vi "_Debug_leer asic y fpga_enlazado.vi"(8 "error in":errorcluster, 11 "Handle":u32) -> (0 "error out":errorcluster, 3 "ftHandle_out":u32)   [LabVIEW 2009]
panel:
  out "Scaler 3 (20,21)":u16 format="%04x"
  out "Scaler 2 (18,19)":u16 format="%04x"
  out "Scaler 1 (16,17)":u16 format="%04x"
  out "Lectura asic (14,15)":u16 format="%04x"
  out "Vent. Sacaler (11,12,13)":u32 format="%06x"
  out "Periodo VGa (9,10)":u16 format="%04x"
  out "Pulse VGa (7,8)":u16 format="%04x"
  out "Ganacia VGA (6)":u8 format="%02x"
  out "adc (4,5)":u16 format="%04x"
  out "Asic (1,2,3)":u32 format="%06x"
  out "DIR 0 (CONFIG)":bool[](array[boolean])
  out "ERROR":bool
  out "UPDATE":bool
  in  "stop":bool
  out "DAC_IB":bool[](array[boolean])
  out "BUFF_ENA":bool
  out "LVDS_ENA1":bool
  out "LVDS_ENA0":bool
  out "MUX_ENA":string
  out "MUX_ENA#":i32
  out "IN 0":bool[](array[boolean])
  out "IN 6":bool[](array[boolean])
  out "IN 5":bool[](array[boolean])
  out "IN 4":bool[](array[boolean])
  out "IN 3":bool[](array[boolean])
  out "IN 2":bool[](array[boolean])
  out "IN 1":bool[](array[boolean])
  out "DAC_MUX#":i32
  out "DAC_MUX":string
  out "TH5":u16 format="%010b"
  out "TH4":u16 format="%010b"
  out "TH3":u16 format="%010b"
  out "TH2":u16 format="%010b"
  out "TH1":u16 format="%010b"
  out "TH0":u16 format="%010b"
  # "start vent. sca\nescribir ganancia\nactualizar pulso\nenable pulso\nstart tx asic\nreset asic\nescribir adc"
  # "IB5\nIB4\nIB3\nIB2\nIB1\nIB0"
  # "Control_byte\nNum bit        Función\n0            \"Escribir\" ADC\n1                      \"INIT_R\" ASIC (reset)\n2                      \"start_tx\" ASIC para configuración ASIC\n3                      \"enable\" para el pulso\n4                      \"actualizar\" para el pulso\n5                      \"Escribir_ganancia\" para configuración ganancia\n6                      \"start\" para apertura ventana temportal scalers"
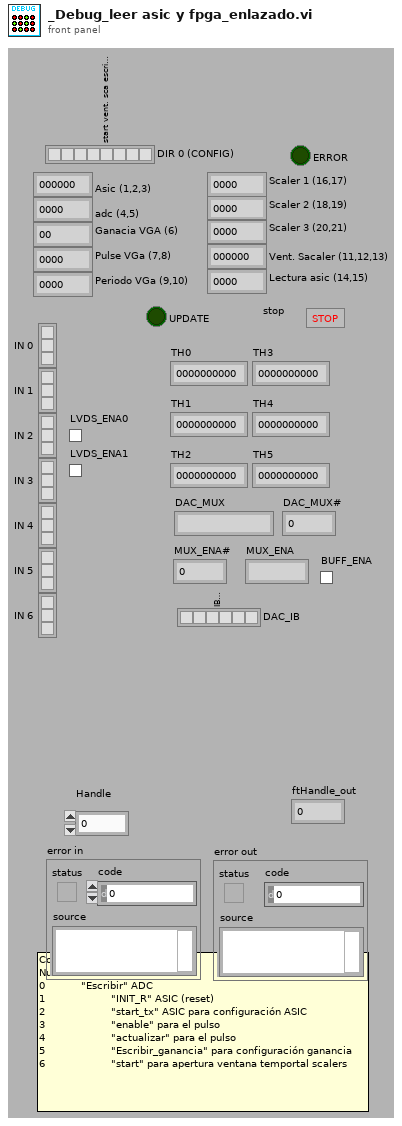
[diagram p1: front panel]
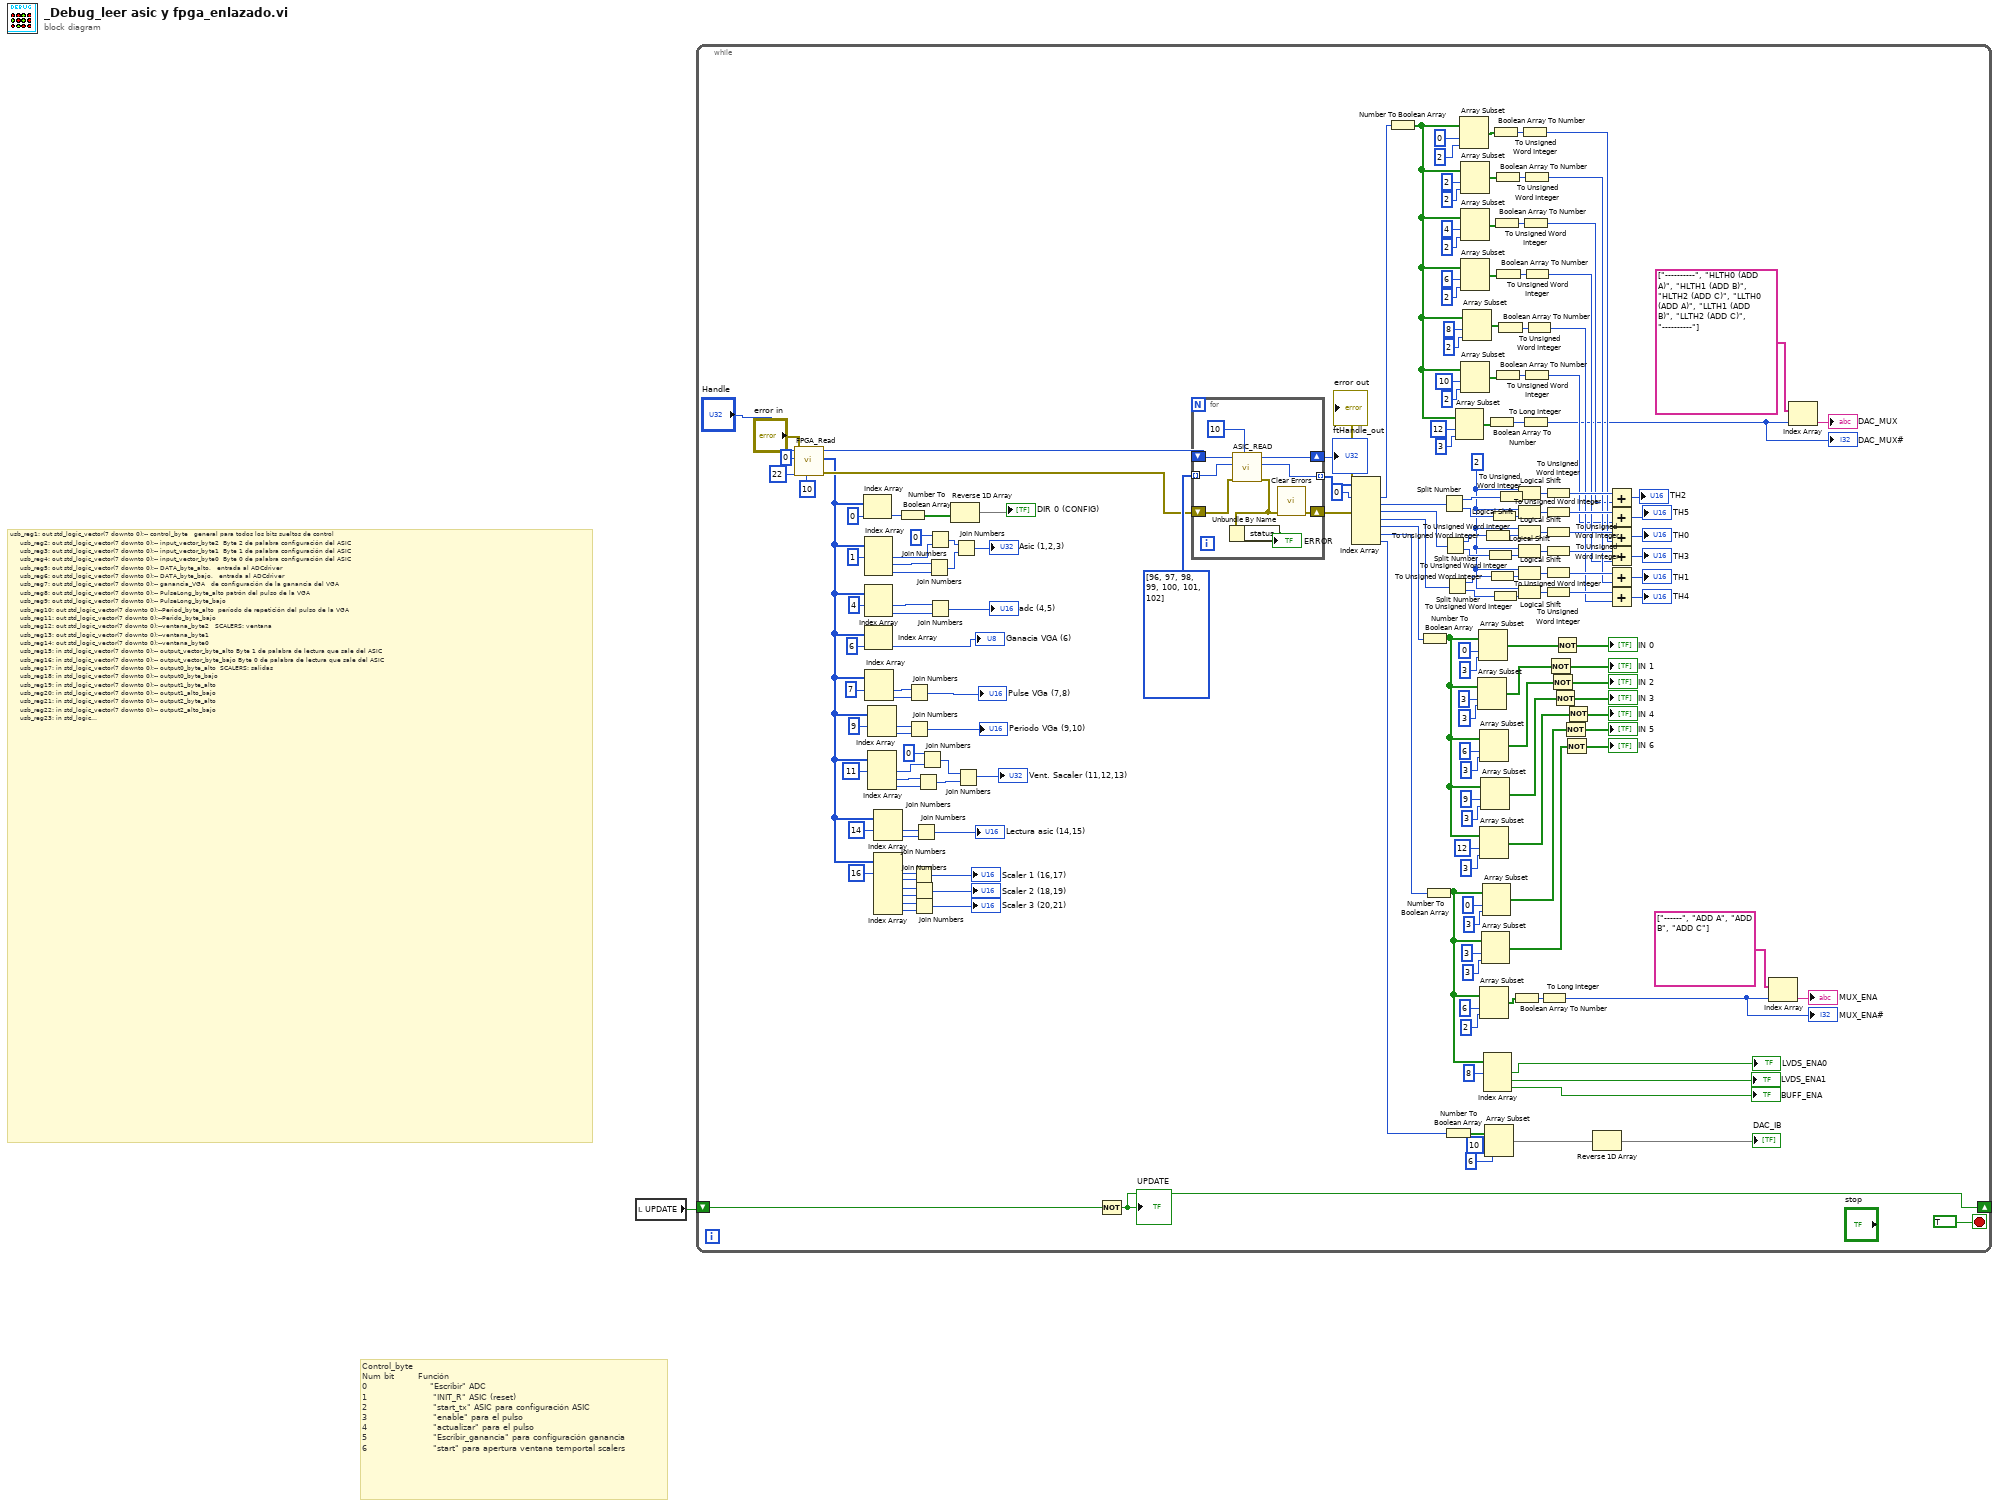
[diagram p0: block diagram]
diagram:
  # "Control_byte\nNum bit        Función\n0                     \"Escribir\" ADC\n1                      \"INIT_R\" ASIC (reset)\n2                      \"start_tx\" ASIC para configuración ASIC\n3                      \"enable\" para el pulso\n4                      \"actualizar\" para el pulso\n5                      \"Escribir_ganancia\" para configuración ganancia\n6                      \"start\" para apertura ventana temportal scalers"
  # "usb_reg1: out std_logic_vector(7 downto 0);-- control_byte\t\t\tgeneral para todos los bits sueltos de control\n\t\t\t  usb_reg2: out std_logic_vector(7 downto 0);-- input_vector_byte2 \tByte 2 de palabra configuración del ASIC\n\t\t\t  usb_reg3: out std_logic_vector(7 downto 0);-- input_vector_byte1 \tByte 1 de palabra configuración del ASIC\n\t\t\t  usb_reg4: out std_logic_vector(7 downto 0);-- input_vector_byte0 \tByte 0 de palabra configuración del ASIC\n\t\t\t  usb_reg5: out std_logic_vector(7 downto 0);-- DATA_byte_alto, \t\tentrada al ADCdriver\n\t\t\t  usb_reg6: out std_logic_vector(7 downto 0);-- DATA_byte_bajo, \t\tentrada al ADCdriver\n\t\t\t  usb_reg7: out std_logic_vector(7 downto 0);-- ganancia_VGA\t\t\tde configuración de la ganancia del VGA\n\t\t\t  usb_reg8: out std_logic_vector(7 downto 0);-- PulseLong_byte_alto\tpatrón del pulso de la VGA\n\t\t\t  usb_reg9: out std_logic_vector(7 downto 0);-- PulseLong_byte_bajo\n\t\t\t  usb_reg10: out std_logic_vector(7 downto 0);--Period_byte_alto\t\tperíodo de repetición del pulso de la VGA\n\t\t\t  usb_reg11: out std_logic_vector(7 downto 0);--Perido_byte_bajo\n\t\t\t  usb_reg12: out std_logic_vector(7 downto 0);--ventana_byte2\t\t\tSCALERS: ventana\n\t\t\t  usb_reg13: out std_logic_vector(7 downto 0);--ventana_byte1\t\n\t\t\t  usb_reg14: out std_logic_vector(7 downto 0);--ventana_byte0\n\t\t\t  usb_reg15: in std_logic_vector(7 downto 0);-- output_vector_byte_alto\tByte 1 de palabra de lectura que sale del ASIC\n\t\t\t  usb_reg16: in std_logic_vector(7 downto 0);-- output_vector_byte_bajo\tByte 0 de palabra de lectura que sale del ASIC\n\t\t\t  usb_reg17: in std_logic_vector(7 downto 0);-- output0_byte_alto\t\tSCALERS: salidas\n\t\t\t  usb_reg18: in std_logic_vector(7 downto 0);-- output0_byte_bajo\n\t\t\t  usb_reg19: in std_logic_vector(7 downto 0);-- output1_byte_alto\n\t\t\t  usb_reg20: in std_logic_vector(7 downto 0);-- output1_alto_bajo \n\t\t\t  usb_reg21: in std_logic_vector(7 downto 0);-- output2_byte_alto \n\t\t\t  usb_reg22: in std_logic_vector(7 downto 0);-- output2_alto_bajo \n\t\t\t  usb_reg23: in std_logic_vector(7 downto 0);-- para el canal_0 del ADCdriver\n\t\t\t  usb_reg24: in std_logic_vector(7 downto 0);\n\t\t\t  usb_reg25: in std_logic_vector(7 downto 0);-- para el canal_1 del ADCdriver\n\t\t\t  usb_reg26: in std_logic_vector(7 downto 0);\n\t\t\t  usb_reg27: in std_logic_vector(7 downto 0);-- para el canal_2 del ADCdriver\n\t\t\t  usb_reg28: in std_logic_vector(7 downto 0);\n\t\t\t  usb_reg29: in std_logic_vector(7 downto 0);-- para el canal_3 del ADCdriver\n\t\t\t  usb_reg30: in std_logic_vector(7 downto 0);\n\t\t\t  usb_reg31: in std_logic_vector(7 downto 0);-- para el canal_4 del ADCdriver\n\t\t\t  usb_reg32: in std_logic_vector(7 downto 0);\n\t\t\t  usb_reg33: in std_logic_vector(7 downto 0);-- para el canal_5 del ADCdriver\n\t\t\t  usb_reg34: in std_logic_vector(7 downto 0);\n\t\t\t  usb_reg35: in std_logic_vector(7 downto 0);-- para el canal_6 del ADCdriver\n\t\t\t  usb_reg36: in std_logic_vector(7 downto 0);\n\t\t\t  usb_reg37: in std_logic_vector(7 downto 0);-- para el canal_7 del ADCdriver\n\t\t\t  usb_reg38: in std_logic_vector(7 downto 0);\n\t\t\t  usb_reg39: in std_logic_vector(7 downto 0);-- para el canal_8 del ADCdriver\n\t\t\t  usb_reg40: in std_logic_vector(7 downto 0);\n\t\t\t  usb_reg41: in std_logic_vector(7 downto 0);-- para el canal_9 del ADCdriver\n\t\t\t  usb_reg42: in std_logic_vector(7 downto 0);\n\t\t\t  usb_reg43: in std_logic_vector(7 downto 0);-- para el canal_10 del ADCdriver\n\t\t\t  usb_reg44: in std_logic_vector(7 downto 0)--;"
  n1 = local read "UPDATE"() -> (w1:bool)
  n2 = while {
    shift-right: [w76] -> _
    shift-left: w1 -> [w14]
    stop <- TRUE stop-if-true
    w176 = i8 2 ("y")
    n3 = call "FPGA_Read.vi"("Espera acceso USB"=u32 10, "error in"="error in", "Numero Bytes"=u8 22, "Dirección base"=u8 0, "ftHandle_in"="Handle") -> ("error out"=w67:errorcluster, "lpBuffer_out"=w26:u8[], "ftHandle_out"=w69:u32)  [unwired: 2 in, 2 out]
    n4 = Index Array(array=w26, index=0) -> (element=w48:u8)
    n5 = Index Array(array=w26, index #1=1 ("index")) -> (element #1=w43:u8, element #2=w44:u8, element #3=w45:u8)  [unwired: 2 in]
    n6 = Index Array(array=w26, index #1=4 ("index")) -> (element #1=w42:u8, element #2=w41:u8)  [unwired: 1 in]
    n7 = Index Array(array=w26, index=6) -> (element=→"Ganacia VGA (6)":u8)
    n8 = Index Array(array=w26, index #1=7 ("index")) -> (element #1=w35:u8, element #2=w36:u8)  [unwired: 1 in]
    n9 = Index Array(array=w26, index #1=9 ("index")) -> (element #1=w33:u8, element #2=w34:u8)  [unwired: 1 in]
    n10 = Index Array(array=w26, index #1=11 ("index")) -> (element #1=w29:u8, element #2=w27:u8, element #3=w28:u8)  [unwired: 2 in]
    n11 = Index Array(array=w26, index #1=14 ("index")) -> (element #1=w25:u8, element #2=w24:u8)  [unwired: 1 in]
    n12 = Index Array(array=w26, index #1=16 ("index")) -> (element #1=w22:u8, element #2=w21:u8, element #3=w19:u8, element #4=w18:u8, element #5=w17:u8, element #6=w16:u8)  [unwired: 5 in]
    n13 = Number To Boolean Array(number=w48) -> (Boolean array=w50:bool[])
    n14 = Join Numbers(hi=w35, lo=w36) -> ((hi.lo)=→"Pulse VGa (7,8)":u16)
    n15 = Join Numbers(hi=w33, lo=w34) -> ((hi.lo)=→"Periodo VGa (9,10)":u16)
    n16 = Join Numbers(hi=w22, lo=w21) -> ((hi.lo)=→"Scaler 1 (16,17)":u16)
    n17 = Join Numbers(hi=w19, lo=w18) -> ((hi.lo)=→"Scaler 2 (18,19)":u16)
    n18 = Join Numbers(hi=w17, lo=w16) -> ((hi.lo)=→"Scaler 3 (20,21)":u16)
    n19 = Join Numbers(hi=w25, lo=w24) -> ((hi.lo)=→"Lectura asic (14,15)":u16)
    n20 = Join Numbers(hi=w27, lo=w28) -> ((hi.lo)=w59:u16)
    n21 = Join Numbers(hi=u8 0, lo=w29) -> ((hi.lo)=w53:u16)
    n22 = Join Numbers(hi=w44, lo=w45) -> ((hi.lo)=w64:u16)
    n23 = Join Numbers(hi=u8 0, lo=w43) -> ((hi.lo)=w63:u16)
    n24 = Join Numbers(hi=w42, lo=w41) -> ((hi.lo)=→"adc (4,5)":u16)
    n25 = Reverse 1D Array(array=w50) -> (reversed array=→"DIR 0 (CONFIG)":bool[])
    n26 = Join Numbers(hi=w63, lo=w64) -> ((hi.lo)=→"Asic (1,2,3)":u32)
    n27 = Join Numbers(hi=w53, lo=w59) -> ((hi.lo)=→"Vent. Sacaler (11,12,13)":u32)
    n28 = Not(x=w14) -> (.not. x?=w76:bool)
    "UPDATE" <- w76
    n29 = for {
      tunnel: u8[] [96, 97, 98, 99, 100, 101, 102] -> [w194] mode=indexing
      tunnel: [w192] -> w186 mode=indexing
      shift-right: [w193] -> w4
      shift-left: w69 -> [w196]
      shift-right: [w191] -> w3
      shift-left: w67 -> [w190]
      n30 = call "ASIC_READ.vi"("Espera acceso USB"=u32 10, "error in"=w190, "Direccion Registro Asic"=w194, "ftHandle_in"=w196) -> ("error out"=w189:errorcluster, "Valor Asic"=w192:u16, "ftHandle_out"=w193:u32)  [unwired: 5 in]
      n31 = Unbundle By Name(w189) -> ("status"=→"ERROR":bool)
      n32 = call <vilib>:"Clear Errors.vi"("error in (no error)"=w189) -> ("error out"=w191:errorcluster)  [unwired: 6 in]
    }
    "ftHandle_out" <- w4
    "error out" <- w3
    n33 = Index Array(array=w186, index #1=0 ("index")) -> (element #1=w118:u16, element #2=w127:u16, element #3=w184:u16, element #4=w183:u16, element #5=w117:u16, element #6=w96:u16, element #7=w80:u16)  [unwired: 6 in]
    n34 = Number To Boolean Array(number=w118) -> (Boolean array=w122:bool[])
    n35 = Number To Boolean Array(number=w117) -> (Boolean array=w105:bool[])
    n36 = Number To Boolean Array(number=w96) -> (Boolean array=w86:bool[])
    n37 = Split Number(x=w127) -> (hi(x)=w182:u8, lo(x)=w181:u8)
    n38 = Split Number(x=w184) -> (hi(x)=w180:u8, lo(x)=w179:u8)
    n39 = Split Number(x=w183) -> (hi(x)=w178:u8, lo(x)=w177:u8)
    n40 = Number To Boolean Array(number=w80) -> (Boolean array=w81:bool[])
    n41 = Array Subset(array=w122, index=12, length=3) -> (w126:bool[])
    n42 = Array Subset(array=w122, index=0, length=2) -> (w173:bool[])
    n43 = Array Subset(array=w122, index=2, length=2) -> (w154:bool[])
    n44 = Array Subset(array=w122, index=4, length=2) -> (w152:bool[])
    n45 = Array Subset(array=w122, index=6, length=2) -> (w150:bool[])
    n46 = Array Subset(array=w122, index=10, length=2) -> (w146:bool[])
    n47 = Array Subset(array=w122, index=8, length=2) -> (w148:bool[])
    n48 = Array Subset(array=w105, index=3, length=3) -> (w104:bool[])
    n49 = Array Subset(array=w105, index=0, length=3) -> (w114:bool[])
    n50 = Array Subset(array=w105, index=6, length=3) -> (w103:bool[])
    n51 = Array Subset(array=w105, index=12, length=3) -> (w101:bool[])
    n52 = Array Subset(array=w86, index=6, length=2) -> (w89:bool[])
    n53 = Array Subset(array=w105, index=9, length=3) -> (w102:bool[])
    n54 = Array Subset(array=w86, index=3, length=3) -> (w94:bool[])
    n55 = Array Subset(array=w86, index=0, length=3) -> (w95:bool[])
    n56 = To Unsigned Word Integer(number=w180) -> (unsigned 16bit integer=w72:u16)
    n57 = Index Array(array=w86, index #1=8 ("index")) -> (element #1=→"LVDS_ENA0":bool, element #2=→"LVDS_ENA1":bool, element #3=→"BUFF_ENA":bool)  [unwired: 2 in]
    n58 = Array Subset(array=w81, index=10, length=6) -> (w77:bool[])
    n59 = To Unsigned Word Integer(number=w179) -> (unsigned 16bit integer=w73:u16)
    n60 = Boolean Array To Number(Boolean array=w126) -> (number=w125:u32)
    n61 = To Unsigned Word Integer(number=w178) -> (unsigned 16bit integer=w74:u16)
    n62 = To Unsigned Word Integer(number=w181) -> (unsigned 16bit integer=w71:u16)
    n63 = To Unsigned Word Integer(number=w177) -> (unsigned 16bit integer=w75:u16)
    n64 = Boolean Array To Number(Boolean array=w173) -> (number=w171:u32)
    n65 = Boolean Array To Number(Boolean array=w152) -> (number=w153:u32)
    n66 = Boolean Array To Number(Boolean array=w154) -> (number=w155:u32)
    n67 = Boolean Array To Number(Boolean array=w146) -> (number=w147:u32)
    n68 = Boolean Array To Number(Boolean array=w150) -> (number=w151:u32)
    n69 = Boolean Array To Number(Boolean array=w148) -> (number=w149:u32)
    n70 = To Unsigned Word Integer(number=w182) -> (unsigned 16bit integer=w70:u16)
    n71 = Boolean Array To Number(Boolean array=w89) -> (number=w88:u32)
    n72 = Logical Shift(y=w176, x=w70) -> (x << y=w172:u16)
    n73 = Logical Shift(y=w176, x=w71) -> (x << y=w169:u16)
    n74 = Logical Shift(y=w176, x=w72) -> (x << y=w145:u16)
    n75 = Logical Shift(y=w176, x=w73) -> (x << y=w144:u16)
    n76 = Logical Shift(y=w176, x=w74) -> (x << y=w143:u16)
    n77 = Logical Shift(y=w176, x=w75) -> (x << y=w142:u16)
    n78 = To Unsigned Word Integer(number=w171) -> (unsigned 16bit integer=w133:u16)
    n79 = To Unsigned Word Integer(number=w153) -> (unsigned 16bit integer=w131:u16)
    n80 = To Long Integer(number=w125) -> (32bit integer=w120:i32)
    "DAC_MUX#" <- w120
    n81 = To Unsigned Word Integer(number=w155) -> (unsigned 16bit integer=w132:u16)
    n82 = To Unsigned Word Integer(number=w147) -> (unsigned 16bit integer=w128:u16)
    n83 = To Unsigned Word Integer(number=w151) -> (unsigned 16bit integer=w130:u16)
    n84 = To Unsigned Word Integer(number=w149) -> (unsigned 16bit integer=w129:u16)
    n85 = To Long Integer(number=w88) -> (32bit integer=w87:i32)
    "MUX_ENA#" <- w87
    n86 = To Unsigned Word Integer(number=w172) -> (unsigned 16bit integer=w170:u16)
    n87 = To Unsigned Word Integer(number=w169) -> (unsigned 16bit integer=w168:u16)
    n88 = To Unsigned Word Integer(number=w145) -> (unsigned 16bit integer=w141:u16)
    n89 = To Unsigned Word Integer(number=w144) -> (unsigned 16bit integer=w140:u16)
    n90 = To Unsigned Word Integer(number=w143) -> (unsigned 16bit integer=w139:u16)
    n91 = To Unsigned Word Integer(number=w142) -> (unsigned 16bit integer=w138:u16)
    n92 = Not(x=w104) -> (.not. x?=→"IN 1":bool[])
    n93 = Not(x=w103) -> (.not. x?=→"IN 2":bool[])
    n94 = Not(x=w102) -> (.not. x?=→"IN 3":bool[])
    n95 = Not(x=w114) -> (.not. x?=→"IN 0":bool[])
    n96 = Not(x=w95) -> (.not. x?=→"IN 5":bool[])
    n97 = Not(x=w94) -> (.not. x?=→"IN 6":bool[])
    n98 = Not(x=w101) -> (.not. x?=→"IN 4":bool[])
    n99 = Reverse 1D Array(array=w77) -> (reversed array=→"DAC_IB":bool[])
    n100 = Add(x=w170, y=w131) -> (x+y=→"TH2":u16)
    n101 = Add(x=w168, y=w128) -> (x+y=→"TH5":u16)
    n102 = Add(x=w141, y=w133) -> (x+y=→"TH0":u16)
    n103 = Add(x=w140, y=w130) -> (x+y=→"TH3":u16)
    n104 = Add(x=w139, y=w132) -> (x+y=→"TH1":u16)
    n105 = Add(x=w138, y=w129) -> (x+y=→"TH4":u16)
    n106 = Index Array(array=string[] ["------", "ADD A", "ADD B", "ADD C"], index=w87) -> (element=→"MUX_ENA":string)
    n107 = Index Array(array=string[] ["----------", "HLTH0 (ADD A)", "HLTH1 (ADD B)", "HLTH2 (ADD C)", "LLTH0 (ADD A)", "LLTH1 (ADD B)", "LLTH2 (ADD C)", "----------"], index=w120) -> (element=→"DAC_MUX":string)
  }
